vi "Knock Write.vi"(0 "Device Inputs":dbl[](array[numeric]), 9 "Controls":T1={"Low Cutoff [Hz]"=-1, "High Cutoff [Hz]"=-1, "Threshold"=-1, "Knock Start [CAD]"=-1, "Knock End [CAD]"=-1, "Reference Start [CAD]"=-1, "Reference End [CAD]"=-1}, 11 "Settings":T2={"Knock Sensor"=[0, 0, 0, 0, 0, 0, 0, 0, 0, 0, 0, 0, 0, 0, 0, 0], "Knock Offset [CAD]"=[0.0, 0.0, 0.0, 0.0, 0.0, 0.0, 0.0, 0.0, 0.0, 0.0, 0.0, 0.0, 0.0, 0.0, 0.0, 0.0]} {"Knock Sensor" items=["Sensor 1", "Sensor 2", "Sensor 3", "Sensor 4", "Sensor 5", "Sensor 6", "Sensor 7", "Sensor 8", "Sensor 9", "Sensor 10", "Sensor 11", "Sensor 12"]}) -> (6 "Knock Settings":T4={"Low Cutoff [Hz]"=5000.0, "High Cutoff [Hz]"=6000.0, "Threshold"=2.0} {"High Cutoff [Hz]" format="%#_6p"; "Low Cutoff [Hz]" format="%#_6p"}, 8 "Knock Windows":T3, 10 "Knock Sensor":i32[](array[ring]) items=["Sensor 1", "Sensor 2", "Sensor 3", "Sensor 4", "Sensor 5", "Sensor 6", "Sensor 7", "Sensor 8", "Sensor 9", "Sensor 10", "Sensor 11", "Sensor 12"], 15 "Knock Offset [CAD]":sgl[](array[numeric]))   [LabVIEW 2016, in "DCM Engine.lvlib"]
uses:
  DCM Engine.lvlib
  Built/DCM Classes Packed/Pharlap/C/DCM-Classes.lvlibp/DCM/Tools/RT/Knock Settings.ctl
  Built/DCM Classes Packed/Pharlap/C/DCM-Classes.lvlibp/FPGA Knock/RevA/RT/Controls/Windows.ctl
  Built/DCM Classes Packed/Pharlap/C/DCM-Classes.lvlibp/DCM/Tools/RT/DCM - RT - Tools.lvlib
  Built/DCM Classes Packed/Pharlap/C/DCM-Classes.lvlibp/FPGA Knock/RevA/RT/Knock - RevA - RT.lvlib
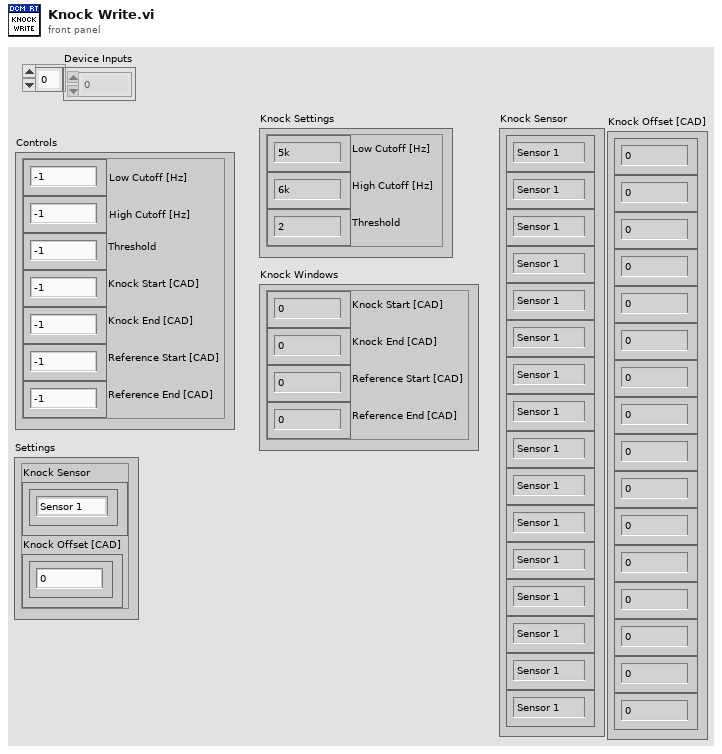
[diagram p1: front panel]
types:
  T1 = cluster{"Low Cutoff [Hz]":i32, "High Cutoff [Hz]":i32, "Threshold":i32, "Knock Start [CAD]":i32, "Knock End [CAD]":i32, "Reference Start [CAD]":i32, "Reference End [CAD]":i32}
  T2 = cluster{"Knock Sensor":i32[], "Knock Offset [CAD]":sgl[]}
  T3 = typedef "DCM-Classes.lvlibp/Knock - RevA - RT.lvlib/Windows.ctl" = cluster{"Knock Start [CAD]":sgl, "Knock End [CAD]":sgl, "Reference Start [CAD]":sgl, "Reference End [CAD]":sgl}
  T4 = typedef "DCM-Classes.lvlibp/DCM - RT - Tools.lvlib/Knock Settings.ctl" = cluster{"Low Cutoff [Hz]":sgl, "High Cutoff [Hz]":sgl, "Threshold":sgl}
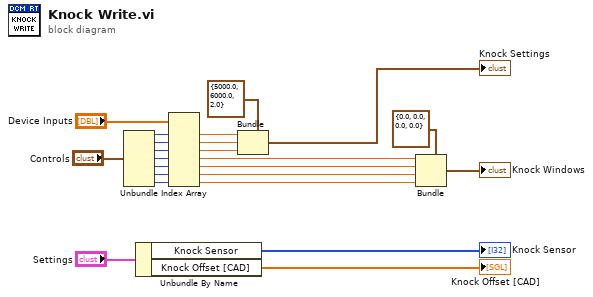
[diagram p0: block diagram]
diagram:
  n1 = Unbundle("Controls") -> ("Low Cutoff [Hz]"=w23:i32, "High Cutoff [Hz]"=w22:i32, "Threshold"=w21:i32, "Knock Start [CAD]"=w4:i32, "Knock End [CAD]"=w3:i32, "Reference Start [CAD]"=w2:i32, "Reference End [CAD]"=w1:i32)
  n2 = Unbundle By Name("Settings") -> ("Knock Sensor"=→"Knock Sensor":i32[], "Knock Offset [CAD]"=→"Knock Offset [CAD]":sgl[])
  n3 = Index Array(array="Device Inputs", index #1=w23, index #2=w22, index #3=w21, index #4=w4, index #5=w3, index #6=w2, index #7=w1) -> (element #1=w18:dbl, element #2=w19:dbl, element #3=w17:dbl, element #4=w13:dbl, element #5=w12:dbl, element #6=w11:dbl, element #7=w10:dbl)
  n4 = Bundle(cluster=T4 {"Low Cutoff [Hz]"=5000.0, "High Cutoff [Hz]"=6000.0, "Threshold"=2.0} ("Knock Settings"), "Low Cutoff [Hz]"=w18, "High Cutoff [Hz]"=w19, "Threshold"=w17) -> (→"Knock Settings":T4)
  n5 = Bundle(cluster=T3 {"Knock Start [CAD]"=0.0, "Knock End [CAD]"=0.0, "Reference Start [CAD]"=0.0, "Reference End [CAD]"=0.0} ("Knock Windows"), "Knock Start [CAD]"=w13, "Knock End [CAD]"=w12, "Reference Start [CAD]"=w11, "Reference End [CAD]"=w10) -> (→"Knock Windows":T3)
